vi "Print VI Panel or Documentation (refnum).vi"(6 "custom contents options":T14 {"list of controls options"."list which controls?" items=["all controls", "connected controls"]}, 7 "layout options":T2={"orientation (unchanged)"=0, "panel scaling for page (unchanged)"=0, "margins"={"override VI margins (false)"=FALSE, "margins (1.00)"={"top"=1.0, "left"=1.0, "right"=1.0, "bottom"=1.0}, "measurement system (default)"=0}, "printer options"={"destination printer name (current)"="", "printing method (unchanged)"=0, "color or monochrome (unchanged)"=0}, "page header options"={"page headers (unchanged)"=0, "page header content options"={"Include VI Name"=TRUE, "Include VI Path"=TRUE, "Include Last Modification Date"=TRUE, "Include Date Printed"=TRUE, "Include Page Number"=TRUE, "Include VI Icon"=TRUE}}} {"page header options"."page headers (unchanged)" items=["Unchanged", "Include page headers", "Do not include page headers"]; "printer options"."color or monochrome (unchanged)" items=["Unchanged", "Color/grayscale", "Monochrome"]; "printer options"."printing method (unchanged)" items=["Unchanged", "Standard", "PostScript", "Bitmap"]; "panel scaling for page (unchanged)" items=["Unchanged", "No Scaling", "Scale front panel to fit"]; "orientation (unchanged)" items=["Unchanged", "portrait", "landscape"]; "margins"."measurement system (default)" items=["Default", "US", "Metric"]; "margins"."margins (1.00)"."right" format="%.2f"; "margins"."margins (1.00)"."bottom" format="%.2f"; "margins"."margins (1.00)"."top" format="%.2f"; "margins"."margins (1.00)"."left" format="%.2f"}, 8 "error in (no error)":errorcluster, 9 "report type (Quick Print)":T1, 10 "contents (complete front panel)":T16 items=["Complete front panel", "Visible portion of front panel", "Icon, description, panel and diagram", "Documentation: Using the panel", "Documentation: Using as a subVI", "Documentation: Complete", "Documentation: Custom"], 11 "VI reference":refnum<vi>) -> (0 "error out":errorcluster, 3 "report out":refnum<class "NI_report.lvclass">)   [LabVIEW 2020, in "NI_ReportGenerationCore.lvlib"]
doc: "Prints a front panel or VI documentation or saves the front panel or VI documentation to a report."
uses:
  <vilib>/Utility/NIReport.llb/NI_ReportGenerationCore.lvlib
  <vilib>/printing/EasyPrintingControls.llb/contents.ctl
  <vilib>/printing/EasyPrintingControls.llb/layout_options.ctl
  <vilib>/printing/EasyPrintingControls.llb/orientation.ctl
  <vilib>/printing/EasyPrintingControls.llb/panel_scaling_for_page.ctl
  <vilib>/printing/EasyPrintingControls.llb/margins.ctl
  <vilib>/printing/EasyPrintingControls.llb/margin_values.ctl
  <vilib>/printing/EasyPrintingControls.llb/measurement_system.ctl
  <vilib>/printing/EasyPrintingControls.llb/printer_options.ctl
  <vilib>/printing/EasyPrintingControls.llb/printing_method.ctl
  <vilib>/printing/EasyPrintingControls.llb/color_or_monochrome.ctl
  <vilib>/printing/EasyPrintingControls.llb/page_header_options.ctl
  <vilib>/printing/EasyPrintingControls.llb/page_headers.ctl
  <vilib>/printing/EasyPrintingControls.llb/page_header_content_options.ctl
  <vilib>/printing/EasyPrintingControls.llb/custom_contents_options.ctl
  <vilib>/printing/EasyPrintingControls.llb/list_which_controls.ctl
  <vilib>/Utility/NIReport.llb/NI_report.lvclass
  <vilib>/Utility/NIReport.llb/Report Type (with Quick Print).ctl
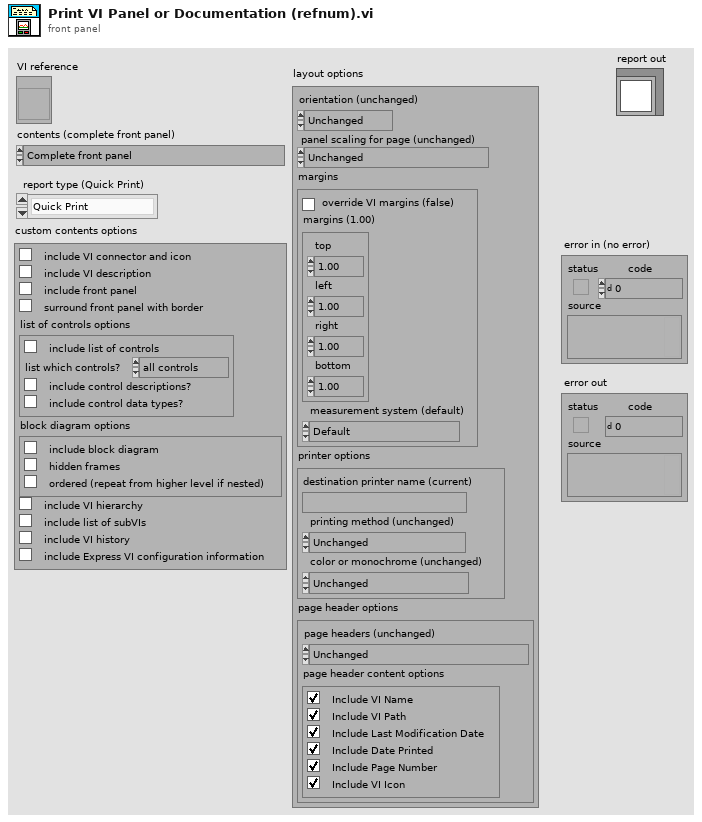
[diagram p1: front panel]
types:
  T1 = typedef "NI_ReportGenerationCore.lvlib/Report Type (with Quick Print).ctl" = enum16{"Quick Print", "HTML", "Word", "Excel"}
  T2 = typedef "NI_ReportGenerationCore.lvlib/layout_options.ctl" = cluster{"orientation (unchanged)":T3, "panel scaling for page (unchanged)":T4, "margins":T5, "printer options":T8, "page header options":T11}
  T3 = typedef "NI_ReportGenerationCore.lvlib/orientation.ctl" = u16
  T4 = typedef "NI_ReportGenerationCore.lvlib/panel_scaling_for_page.ctl" = u16
  T5 = typedef "NI_ReportGenerationCore.lvlib/margins.ctl" = cluster{"override VI margins (false)":bool, "margins (1.00)":T6, "measurement system (default)":T7}
  T6 = typedef "NI_ReportGenerationCore.lvlib/margin_values.ctl" = cluster{"top":dbl, "left":dbl, "right":dbl, "bottom":dbl}
  T7 = typedef "NI_ReportGenerationCore.lvlib/measurement_system.ctl" = u16
  T8 = typedef "NI_ReportGenerationCore.lvlib/printer_options.ctl" = cluster{"destination printer name (current)":string, "printing method (unchanged)":T9, "color or monochrome (unchanged)":T10}
  T9 = typedef "NI_ReportGenerationCore.lvlib/printing_method.ctl" = u16
  T10 = typedef "NI_ReportGenerationCore.lvlib/color_or_monochrome.ctl" = u16
  T11 = typedef "NI_ReportGenerationCore.lvlib/page_header_options.ctl" = cluster{"page headers (unchanged)":T12, "page header content options":T13}
  T12 = typedef "NI_ReportGenerationCore.lvlib/page_headers.ctl" = u16
  T13 = typedef "NI_ReportGenerationCore.lvlib/page_header_content_options.ctl" = cluster{"Include VI Name":bool, "Include VI Path":bool, "Include Last Modification Date":bool, "Include Date Printed":bool, "Include Page Number":bool, "Include VI Icon":bool}
  T14 = typedef "NI_ReportGenerationCore.lvlib/custom_contents_options.ctl" = cluster{"include VI connector and icon":bool, "include VI description":bool, "include front panel":bool, "surround front panel with border":bool, "list of controls options":cluster{"include list of controls":bool, "list which controls?":T15, "include control descriptions?":bool, "include control data types?":bool}, "block diagram options":cluster{"include block diagram":bool, "hidden frames":bool, "ordered (repeat from higher level if nested)":bool}, "include VI hierarchy":bool, "include list of subVIs":bool, "include VI history":bool, "include Express VI configuration information":bool}
  T15 = typedef "NI_ReportGenerationCore.lvlib/list_which_controls.ctl" = u16
  T16 = typedef "NI_ReportGenerationCore.lvlib/contents.ctl" = u16
  T17 = enum16{"Standard Report", "HTML", "Word", "Excel"}
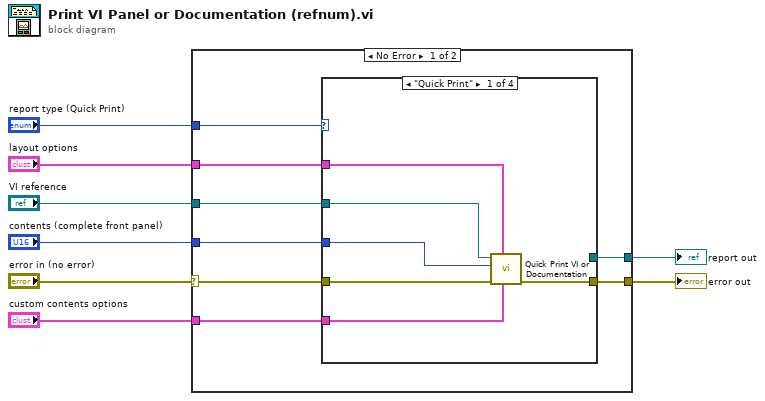
[diagram p0: block diagram]
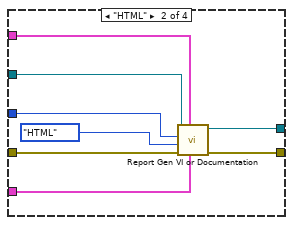
[diagram p2: hidden frame]
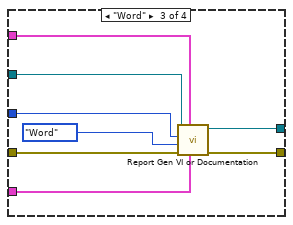
[diagram p3: hidden frame]
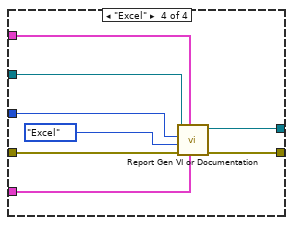
[diagram p4: hidden frame]
diagram:
  n1 = case shown="No Error" "error in (no error)" {
    selector: "error in (no error)" -> [w15 w47]
    tunnel: [w16 w47] -> w7
    tunnel: [w14 _] -> w6
    tunnel: "layout options" -> [w13 _]
    tunnel: "VI reference" -> [w12 _]
    tunnel: "report type (Quick Print)" -> [w11 _]
    tunnel: "contents (complete front panel)" -> [w10 _]
    tunnel: "custom contents options" -> [w9 _]
    frame No Error {
      n2 = case shown="\"Quick Print\"" w11 {
        tunnel: [w21 w24 w32 w40] -> w16
        tunnel: w12 -> [w17 w23 w31 w39]
        tunnel: w10 -> [w20 w29 w36 w44]
        tunnel: w13 -> [w19 w30 w37 w45]
        tunnel: w9 -> [w18 w27 w34 w42]
        tunnel: w15 -> [w22 w28 w35 w41]
        tunnel: [_ w26 w38 w46] -> w14
        frame "Quick Print" {
          n3 = call <vilib>:"Quick Print VI or Documentation.vi"("custom contents options"=w18, "layout options"=w19, "error in (no error)"=w22, "contents (complete front panel)"=w20, "VI reference"=w17) -> ("error out"=w21:errorcluster)  [unwired: 6 in]
        }
        frame "HTML" {
          n4 = call <vilib>:"Report Gen VI or Documentation.vi"("custom contents options"=w27, "layout options"=w30, "error in (no error)"=w28, "report type"=T17."HTML", "contents (complete front panel)"=w29, "VI reference"=w23) -> ("error out"=w24:errorcluster, "report out"=w26:refnum<class "NI_report.lvclass">)  [unwired: 4 in]
        }
        frame "Word" {
          n5 = call <vilib>:"Report Gen VI or Documentation.vi"("custom contents options"=w34, "layout options"=w37, "error in (no error)"=w35, "report type"=T17."Word", "contents (complete front panel)"=w36, "VI reference"=w31) -> ("error out"=w32:errorcluster, "report out"=w38:refnum<class "NI_report.lvclass">)  [unwired: 4 in]
        }
        frame "Excel" {
          n6 = call <vilib>:"Report Gen VI or Documentation.vi"("custom contents options"=w42, "layout options"=w45, "error in (no error)"=w41, "report type"=T17."Excel", "contents (complete front panel)"=w44, "VI reference"=w39) -> ("error out"=w40:errorcluster, "report out"=w46:refnum<class "NI_report.lvclass">)  [unwired: 4 in]
        }
      }
    }
    frame Error {
    }
  }
  "error out" <- w7
  "report out" <- w6
